vi "JSON to array.vi"(8 "error in (no error)":errorcluster, 11 "JSON Data In":string) -> (0 "error out":errorcluster, 2 "values":string[](array[string]), 3 "names":string[][](array[string]))   [LabVIEW 2019, in "Userlib.lvlib"]
uses:
  Userlib.lvlib
  <vilib>/JDP Science/JSONtext/String Subset.vi
  <vilib>/JDP Science/JSONtext/support/Strip Quotes and Unescape.vi
  <vilib>/JDP Science/JSONtext/Parsing/Parse Full Path or Item Name.vi
  <vilib>/JDP Science/JSONtext/Offset/Find Item Locations by Path.vi
  <vilib>/JDP Science/JSONtext/support/Unescape JSON string.vi
  <vilib>/JDP Science/JSONtext/JSONtext.lvlib
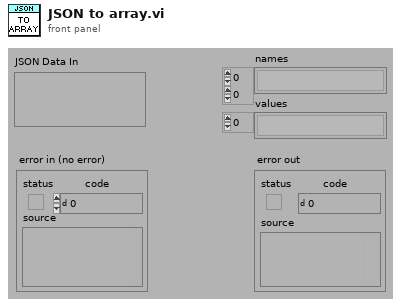
[diagram p1: front panel]
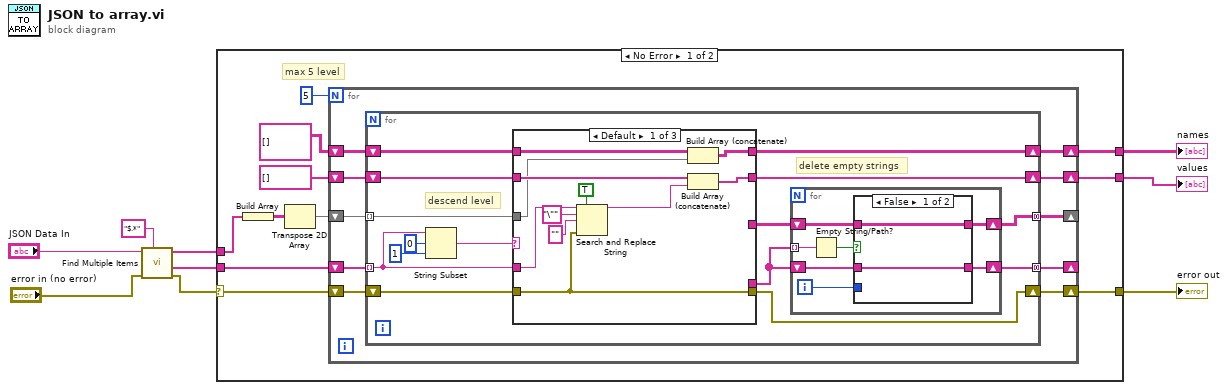
[diagram p0: block diagram]
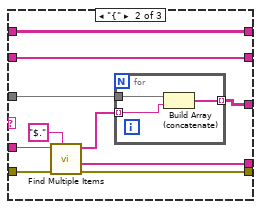
[diagram p2: hidden frame]
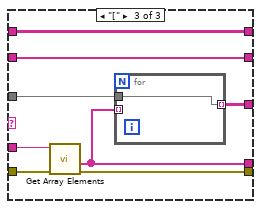
[diagram p3: hidden frame]
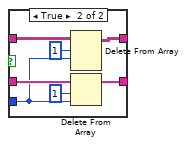
[diagram p4: hidden frame]
diagram:
  n1 = call <vilib>:"Find Multiple Items.vi"("$Path or Item Name"="$.*", "error in (no error)"="error in (no error)", "JSON"="JSON Data In") -> ("error out"=w4:errorcluster, "<JSON>"=w7:string[], "Item Names"=w6:string[])  [unwired: 5 in, 1 out]
  n2 = case shown="No Error" w4 {
    selector: w4 -> [w17 w95]
    tunnel: w7 -> [w19 _]
    tunnel: w6 -> [w12 _]
    tunnel: [w15 w95] -> w1
    tunnel: [w14 _] -> w3
    tunnel: [w13 _] -> w2
    frame No Error {
      # "max 5 level"
      n3 = Build Array(w12) -> (w11:string[][])
      n4 = Transpose 2D Array(2D array=w11) -> (transposed array=w10:string[][])
      n5 = for {
        N: 5 -> [_]
        shift-right: [w29] -> w13
        shift-left: string[] [] -> [w30]
        shift-right: [w26] -> _
        shift-left: w10 -> [w28]
        shift-right: [w25] -> _
        shift-left: w19 -> [w27]
        shift-right: [w23] -> w15
        shift-left: w17 -> [w24]
        shift-right: [w22] -> w14
        shift-left: string[][] [] -> [w21]
        n6 = for {
          shift-right: [w42] -> w29
          shift-left: w30 -> [w45]
          tunnel: [w38] -> w26 mode=concatenating
          tunnel: [w37] -> w25 mode=concatenating
          tunnel: w28 -> [w41] mode=indexing
          tunnel: w27 -> [w40] mode=indexing
          shift-right: [w34] -> w23
          shift-left: w24 -> [w35]
          shift-right: [w33] -> w22
          shift-left: w21 -> [w32]
          # "delete empty strings"
          # "descend level"
          n7 = String Subset(string=w40, offset (0)=0, length (rest)=1 ("length (rest)")) -> (substring=w31:string)
          n8 = case shown="Default" w31 {
            tunnel: w40 -> [w51 w64 w73]
            tunnel: w41 -> [w52 w63 w76]
            tunnel: w45 -> [w56 w66 w77]
            tunnel: [w55 w66 w77] -> w42
            tunnel: [_ w62 w70] -> w39
            tunnel: [_ w57 w75] -> w36
            tunnel: w35 -> [w48 w60 w72]
            tunnel: [w48 w59 w71] -> w34
            tunnel: [w53 w58 w74] -> w33
            tunnel: w32 -> [w54 w58 w74]
            frame Default {
              n9 = Search and Replace String(replace all?=TRUE ("replace all? (F)"), input string=w51, search string="\"", replace string="" ("replace string (\"\")"), error in=w48) -> (result string=w47:string)  [unwired: 3 in, 3 out]
              n10 = Build Array (concatenate)(w54, w52) -> (w53:string[][])
              n11 = Build Array (concatenate)(w56, w47) -> (w55:string[])
            }
            frame "{" {
              n12 = call <vilib>:"Find Multiple Items.vi"("$Path or Item Name"="$.", "error in (no error)"=w60, "JSON"=w64) -> ("error out"=w59:errorcluster, "<JSON>"=w62:string[], "Item Names"=w61:string[])  [unwired: 5 in, 1 out]
              n13 = for {
                tunnel: w61 -> [w67] mode=indexing
                tunnel: w63 -> [w68]
                tunnel: [w69] -> w57 mode=indexing
                n14 = Build Array (concatenate)(w68, w67) -> (w69:string[])
              }
            }
            frame "[" {
              n15 = call <vilib>:"Get Array Elements.vi"("error in (no error)"=w72, "JSON"=w73) -> ("error out"=w71:errorcluster, "<JSON>"=w70:string[])  [unwired: 7 in, 1 out]
              n16 = for {
                tunnel: w76 -> [w78]
                tunnel: [w78] -> w75 mode=indexing
                tunnel: w70 -> [_] mode=indexing
              }
            }
          }
          n17 = for {
            shift-right: [w80] -> w38
            shift-left: w36 -> [w82]
            shift-right: [w79] -> w37
            shift-left: w39 -> [w81]
            tunnel: w39 -> [w85] mode=indexing
            i -> [w83]
            n18 = Empty String/Path?(string/path=w85) -> (empty?=w84:bool)
            n19 = case shown="False" w84 {
              tunnel: w83 -> [_ w88]
              tunnel: w82 -> [w87 w94]
              tunnel: w81 -> [w86 w91]
              tunnel: [w87 w90] -> w80
              tunnel: [w86 w89] -> w79
              frame False {
              }
              frame True {
                n20 = Delete From Array(array=w94, length=1, index (row)=w88) -> (array with subset deleted=w90:string[][])  [unwired: 1 in, 1 out]
                n21 = Delete From Array(array=w91, length=1, index=w88) -> (array with subset deleted=w89:string[])  [unwired: 1 out]
              }
            }
          }
        }
      }
    }
    frame Error {
    }
  }
  "error out" <- w1
  "names" <- w3
  "values" <- w2
